vi "Handle Heater DC.vi"(9 "DC":u8[](array[numeric]), 10 "CVT Session":T1, 11 "nData in":refnum<class "SOAP Data.lvclass">) -> (3 "nData out":refnum<class "SOAP Data.lvclass">)   [LabVIEW 2017, in "Controller.lvlib" / "SOAP Data.lvclass"]
uses:
  SOAP Data.lvclass
  <vilib>/MSR Consulting, LLC/General Reuse/Session APIs/_Session Fwk/Typedefs/Session Handle.ctl
  <vilib>/MSR Consulting, LLC/General Reuse/Session APIs/_Session Fwk/Session - Root.lvclass
  SOAP Data.lvclass/SOAP Data.ctl
  Heater Data/Heater Data.lvclass
  <vilib>/MSR Consulting, LLC/General Reuse/Session APIs/CVT/CVT.lvclass
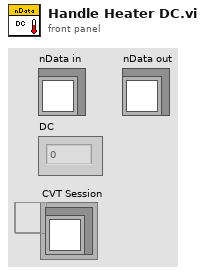
[diagram p1: front panel]
types:
  T1 = typedef "Session - Root.lvclass/Session Handle.ctl" = refnum<data-value>
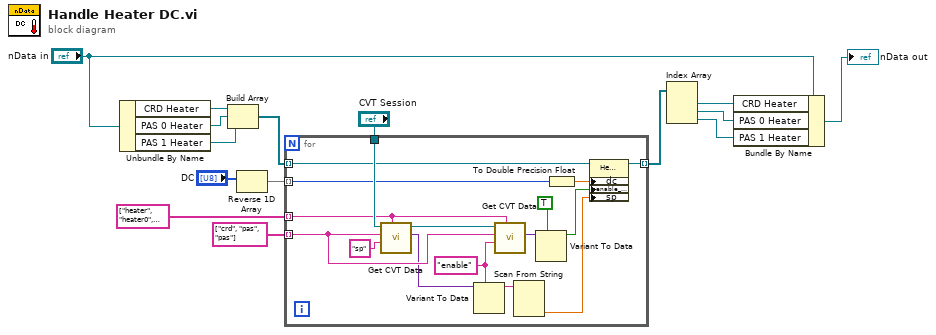
[diagram p0: block diagram]
diagram:
  n1 = Unbundle By Name("nData in") -> ("CRD Heater"=w13:refnum<class "Heater Data.lvclass">, "PAS 0 Heater"=w12:refnum<class "Heater Data.lvclass">, "PAS 1 Heater"=w11:refnum<class "Heater Data.lvclass">)
  n2 = Build Array(w13, w12, w11) -> (w10:refnum<class "Heater Data.lvclass">[])
  n3 = Reverse 1D Array(array="DC") -> (reversed array=w14:u8[])
  n4 = for {
    tunnel: string[] ["crd", "pas", "pas"] -> [w27] mode=indexing
    tunnel: string[] ["heater", "heater0", "heater1"] -> [w28] mode=indexing
    tunnel: "CVT Session" -> [w31]
    tunnel: w14 -> [w17] mode=indexing
    tunnel: w10 -> [w21] mode=indexing
    tunnel: [w18] -> w6 mode=indexing
    w25 = "enable" ("Variable")
    n5 = call <vilib>:"Get CVT Data.vi"("Subgroup"=w28, "Variable"="sp", "Group"=w27, "CVT Session In"=w31) -> ("Data Out"=w26:variant, "CVT Session Out"=w29:T1)  [unwired: 4 in, 2 out]
    n6 = Variant To Data(type=w25, Variant=w26) -> (data=w24:string)  [unwired: 1 in, 1 out]
    n7 = call <vilib>:"Get CVT Data.vi"("Subgroup"=w28, "Variable"=w25, "Group"=w27, "CVT Session In"=w29) -> ("Data Out"=w23:variant)  [unwired: 4 in, 3 out]
    n8 = Scan From String(input string=w24) -> (output 1=w19:dbl)  [unwired: 4 in, 3 out]
    n9 = Variant To Data(type=TRUE, Variant=w23) -> (data=w20:bool)  [unwired: 1 in, 1 out]
    n10 = To Double Precision Float(number=w17) -> (double precision float=w16:dbl)
    n11 = property class="Heater Data"(reference=w21, "dc"=w16, "enable_ctl"=w20, "sp"=w19) -> (reference out=w18:refnum<class "Heater Data.lvclass">)  [unwired: 1 in, 1 out]
  }
  n12 = Index Array(array=w6) -> (element #1=w4:refnum<class "Heater Data.lvclass">, element #2=w3:refnum<class "Heater Data.lvclass">, element #3=w2:refnum<class "Heater Data.lvclass">)  [unwired: 3 in]
  n13 = Bundle By Name(cluster="nData in", "CRD Heater"=w4, "PAS 0 Heater"=w3, "PAS 1 Heater"=w2) -> (→"nData out":refnum<class "SOAP Data.lvclass">)
